vi "PicoScope4000aStartStreaming.vi"(0 "error in":errorcluster, 1 "handle in":i16, 4 "Enabled array":i16[](array[numeric]), 5 "Acquisition Settings":T1 {"Time Units" items=["Nanoseconds (ns)", "Microseconds (us)", "Milliseconds (ms)", "Seconds (s)"]; "Down-Sample Mode" items=["None", "Aggregate", "Decimate", "Average"]}) -> (6 "Channel A":i16[](array[numeric]), 7 "Channel E":i16[](array[numeric]), 8 "Channel B":i16[](array[numeric]), 9 "Channel F":i16[](array[numeric]), 10 "Channel C":i16[](array[numeric]), 11 "Channel G":i16[](array[numeric]), 12 "Channel D":i16[](array[numeric]), 13 "Channel H":i16[](array[numeric]), 14 "error out":errorcluster, 15 "handle out":i16, 18 "Sample Interval":u32)   [LabVIEW 2009]
doc: "This VI starts the oscilloscope streaming. It outputs arrays that will contain samples once PicoScope3000aGetStreamingValues.vi has returned."
uses:
  ps4000aWrap.dll
  PS4000a.dll
panel:
  out "Channel H Min":i16[](array[numeric])
  out "Channel G Min":i16[](array[numeric])
  out "Channel F Min":i16[](array[numeric])
  out "Channel E Min":i16[](array[numeric])
  out "Channel D Min":i16[](array[numeric])
  out "Channel C Min":i16[](array[numeric])
  out "Channel B Min":i16[](array[numeric])
  out "Channel A Min":i16[](array[numeric])
  # "Overview Buffer Size is the size of the temporary buffers used to\nstore data before returning it to the application."
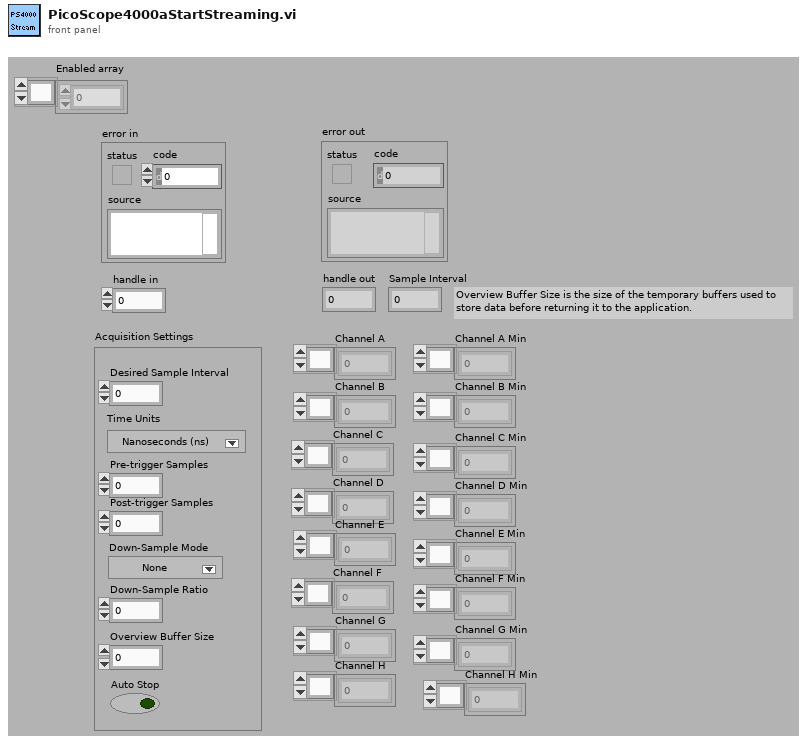
[diagram p1: front panel]
types:
  T1 = cluster{"Auto Stop":bool, "Desired Sample Interval":u32, "Pre-trigger Samples":u32, "Post-trigger Samples":u32, "Down-Sample Ratio":u32, "Down-Sample Mode":i32, "Overview Buffer Size":u32, "Time Units":u32}
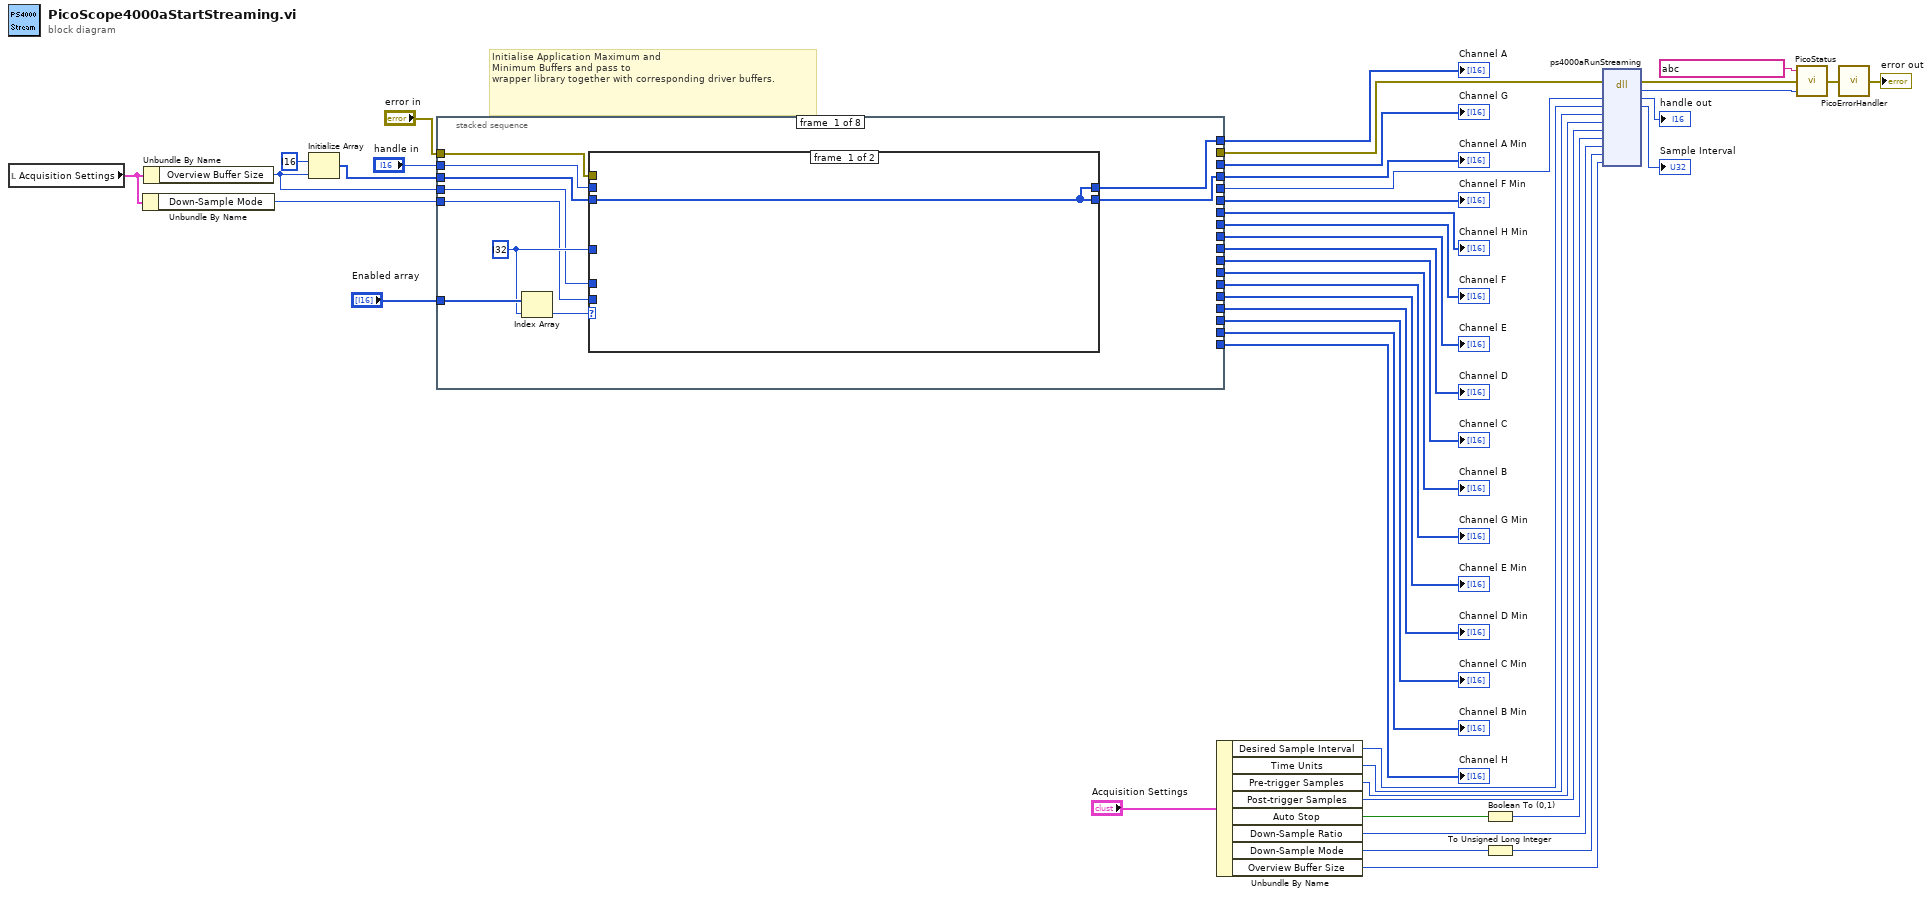
[diagram p0: block diagram]
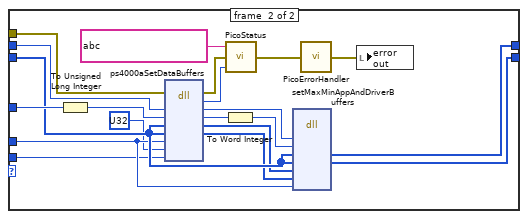
[diagram p2: hidden frame]
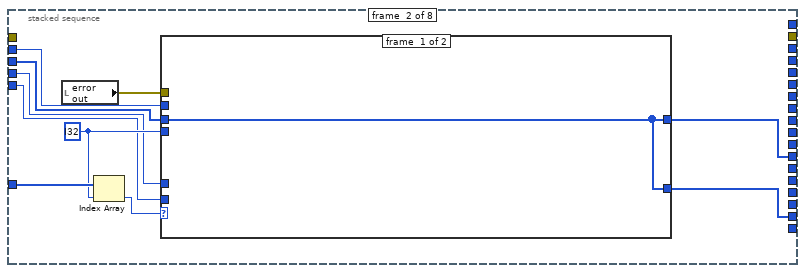
[diagram p3: hidden frame]
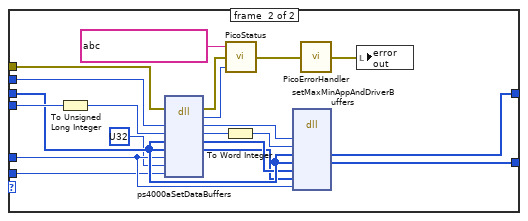
[diagram p4: hidden frame]
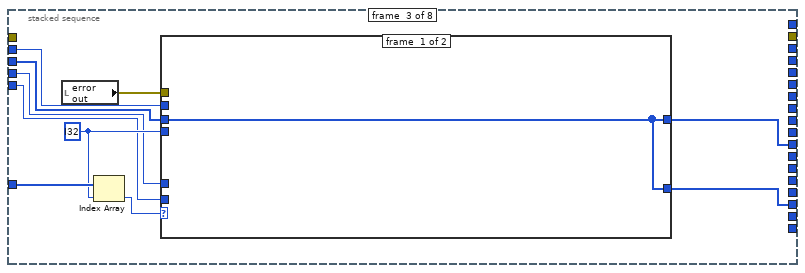
[diagram p5: hidden frame]
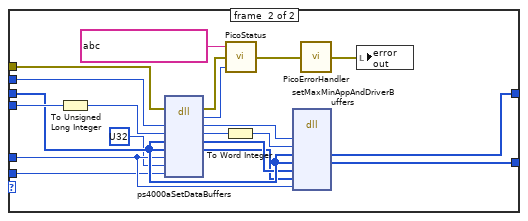
[diagram p6: hidden frame]
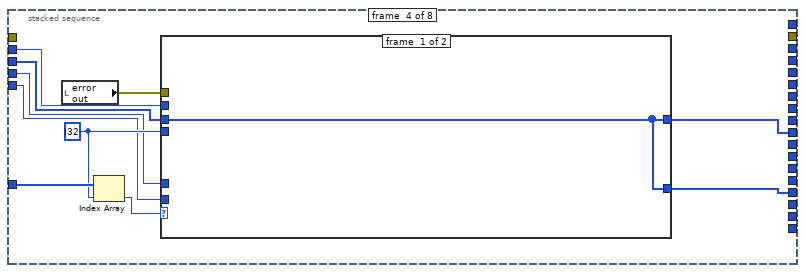
[diagram p7: hidden frame]
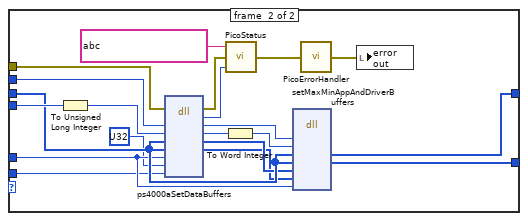
[diagram p8: hidden frame]
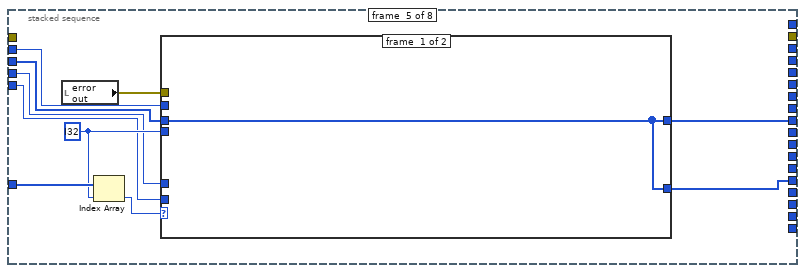
[diagram p9: hidden frame]
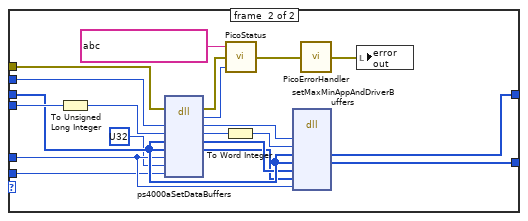
[diagram p10: hidden frame]
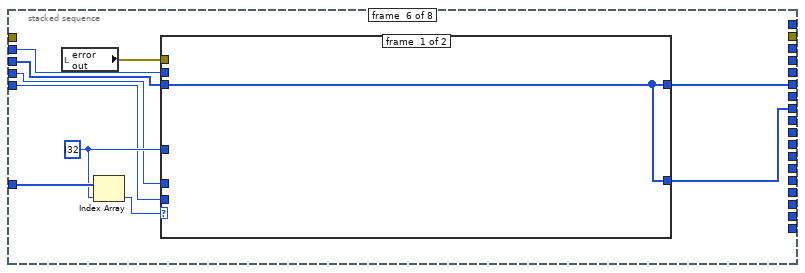
[diagram p11: hidden frame]
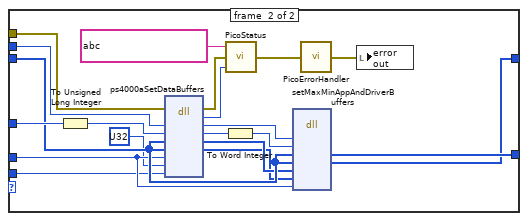
[diagram p12: hidden frame]
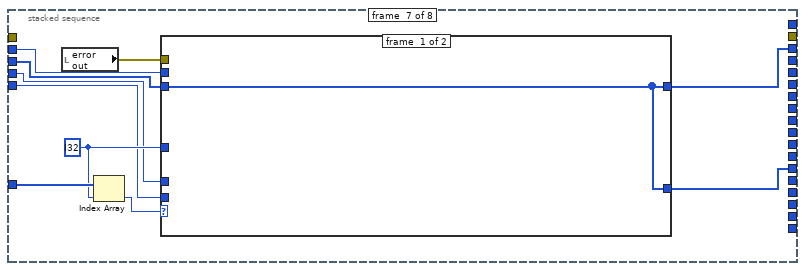
[diagram p13: hidden frame]
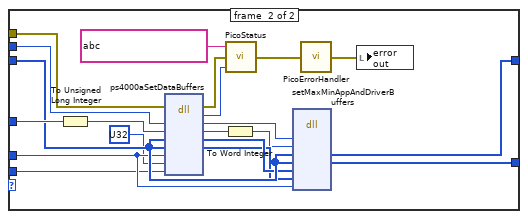
[diagram p14: hidden frame]
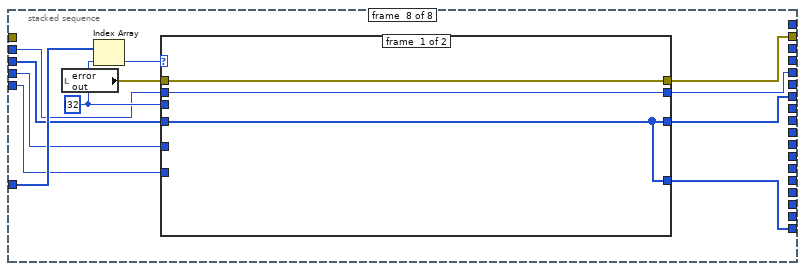
[diagram p15: hidden frame]
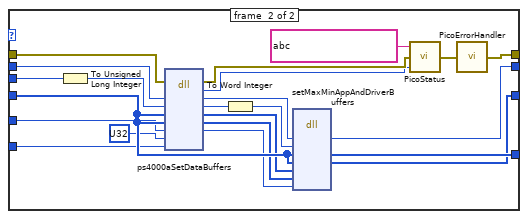
[diagram p16: hidden frame]
diagram:
  # "Initialise Application Maximum and\nMinimum Buffers and pass to \nwrapper library together with corresponding driver buffers."
  n1 = local read "Acquisition Settings"() -> (w31:T1)
  n2 = Unbundle By Name(w31) -> ("Down-Sample Mode"=w24:i32)
  n3 = Unbundle By Name(w31) -> ("Overview Buffer Size"=w22:u32)
  n4 = Initialize Array(i16 ? ("element"), w22) -> (w25:i16[])
  n5 = stacked-sequence {
    tunnel: "Enabled array" -> [w53 w84 w115 w146 w177 w208 w239 w272]
    tunnel: w25 -> [w51 w82 w113 w144 w175 w206 w237 w270]
    tunnel: "error in" -> [w50 _ _ _ _ _ _ _]
    tunnel: [w49 _ _ _ _ _ _ _] -> w16
    tunnel: [w48 _ _ _ _ _ _ _] -> w15
    tunnel: w22 -> [w47 w81 w112 w143 w174 w205 w236 w269]
    tunnel: w24 -> [w46 w80 w111 w142 w173 w204 w235 w268]
    tunnel: "handle in" -> [w45 w79 w110 w141 w172 w203 w234 w267]
    tunnel: [_ w78 _ _ _ _ _ _] -> w9
    tunnel: [_ w77 _ _ _ _ _ _] -> w14
    tunnel: [_ _ w108 _ _ _ _ _] -> w8
    tunnel: [_ _ w107 _ _ _ _ _] -> w13
    tunnel: [_ _ _ w139 _ _ _ _] -> w7
    tunnel: [_ _ _ w138 _ _ _ _] -> w11
    tunnel: [_ _ _ _ w170 _ _ _] -> w6
    tunnel: [_ _ _ _ w169 _ _ _] -> w12
    tunnel: [_ _ _ _ _ w201 _ _] -> w4
    tunnel: [_ _ _ _ _ w200 _ _] -> w5
    tunnel: [_ _ _ _ _ _ w232 _] -> w2
    tunnel: [_ _ _ _ _ _ w231 _] -> w3
    tunnel: [_ _ _ _ _ _ _ w265] -> w1
    tunnel: [_ _ _ _ _ _ _ w264] -> w10
    tunnel: [_ _ _ _ _ _ _ w263] -> w18
    tunnel: [_ _ _ _ _ _ _ w262] -> w17
    frame #0 {
      w52 = i32 ? ("index")
      n6 = Index Array(array=w53, index=w52) -> (element=w54:i16)
      n7 = case shown="1" w54 {
        tunnel: w52 -> [_ w75]
        tunnel: w51 -> [w55 w72]
        tunnel: w50 -> [_ w73]
        tunnel: [w55 w63] -> w49
        tunnel: [w55 w62] -> w48
        tunnel: w47 -> [_ w60]
        tunnel: w46 -> [_ w58]
        tunnel: w45 -> [_ w56]
        frame #0 {
        }
        frame #1 {
          n8 = To Unsigned Long Integer(number=w75) -> (unsigned 32bit integer=w74:u32)
          n9 = dll-call lib="PS4000a.dll" fn="ps4000aSetDataBuffers" ("ps3000.dll:_ps3000_open_unit@0")(error in=w73, "handle"=w56, "channel"=w74, "bufferMax"=w72, "bufferMin"=w72, "bufferLth"=w60, "segmentIndex"=u32 ?, "mode"=w58) -> (error out=w66:errorcluster, "PICO_STATUS"=w65:u32, "handle"=w69:i16, "channel"=w68:u32, "bufferMax"=w71:i16[], "bufferMin"=w70:i16[])  [unwired: 5 in, 1 out]
          n10 = To Word Integer(number=w68) -> (16bit integer=w67:i16)
          n11 = call "PicoStatus.vi"("PICO STATUS"=w65, "error in"=w66, "source"=string ?) -> ("error out"=w61:errorcluster)
          n12 = dll-call lib="ps4000aWrap.dll" fn="setMaxMinAppAndDriverBuffers" label="setMaxMinAppAndDriverBuffers\n(Channel A)"("handle"=w69, "channel"=w67, "appMaxBuffer"=w72, "appMinBuffer"=w72, "driverMaxBuffer"=w71, "driverMinBuffer"=w70, "bufferLength"=w60) -> ("appMaxBuffer"=w63:i16[], "appMinBuffer"=w62:i16[])  [unwired: 9 in, 2 out]
          n13 = call "PicoErrorHandler.vi"("error in"=w61) -> ("error out"=w57:errorcluster)
          n14 = local write "error out"(w57) -> ()
        }
      }
    }
    frame #1 {
      w83 = i32 ? ("index")
      n15 = local read "error out"() -> (w76:errorcluster)
      n16 = Index Array(array=w84, index=w83) -> (element=w85:i16)
      n17 = case shown="1" w85 {
        tunnel: w83 -> [_ w106]
        tunnel: w82 -> [w86 w103]
        tunnel: w76 -> [_ w104]
        tunnel: [w86 w94] -> w78
        tunnel: [w86 w93] -> w77
        tunnel: w81 -> [_ w91]
        tunnel: w80 -> [_ w89]
        tunnel: w79 -> [_ w87]
        frame #0 {
        }
        frame #1 {
          n18 = To Unsigned Long Integer(number=w106) -> (unsigned 32bit integer=w105:u32)
          n19 = dll-call lib="PS4000a.dll" fn="ps4000aSetDataBuffers" ("ps3000.dll:_ps3000_open_unit@0")(error in=w104, "handle"=w87, "channel"=w105, "bufferMax"=w103, "bufferMin"=w103, "bufferLth"=w91, "segmentIndex"=u32 ?, "mode"=w89) -> (error out=w97:errorcluster, "PICO_STATUS"=w96:u32, "handle"=w100:i16, "channel"=w99:u32, "bufferMax"=w102:i16[], "bufferMin"=w101:i16[])  [unwired: 5 in, 1 out]
          n20 = To Word Integer(number=w99) -> (16bit integer=w98:i16)
          n21 = call "PicoStatus.vi"("PICO STATUS"=w96, "error in"=w97, "source"=string ?) -> ("error out"=w92:errorcluster)
          n22 = dll-call lib="ps4000aWrap.dll" fn="setMaxMinAppAndDriverBuffers" label="setMaxMinAppAndDriverBuffers\n(Channel B)"("handle"=w100, "channel"=w98, "appMaxBuffer"=w103, "appMinBuffer"=w103, "driverMaxBuffer"=w102, "driverMinBuffer"=w101, "bufferLength"=w91) -> ("appMaxBuffer"=w94:i16[], "appMinBuffer"=w93:i16[])  [unwired: 9 in, 2 out]
          n23 = call "PicoErrorHandler.vi"("error in"=w92) -> ("error out"=w88:errorcluster)
          n24 = local write "error out"(w88) -> ()
        }
      }
    }
    frame #2 {
      w114 = i32 ? ("index")
      n25 = local read "error out"() -> (w109:errorcluster)
      n26 = Index Array(array=w115, index=w114) -> (element=w116:i16)
      n27 = case shown="1" w116 {
        tunnel: w114 -> [_ w137]
        tunnel: w113 -> [w117 w134]
        tunnel: w109 -> [_ w135]
        tunnel: [w117 w125] -> w108
        tunnel: [w117 w124] -> w107
        tunnel: w112 -> [_ w122]
        tunnel: w111 -> [_ w120]
        tunnel: w110 -> [_ w118]
        frame #0 {
        }
        frame #1 {
          n28 = To Unsigned Long Integer(number=w137) -> (unsigned 32bit integer=w136:u32)
          n29 = dll-call lib="PS4000a.dll" fn="ps4000aSetDataBuffers" ("ps3000.dll:_ps3000_open_unit@0")(error in=w135, "handle"=w118, "channel"=w136, "bufferMax"=w134, "bufferMin"=w134, "bufferLth"=w122, "segmentIndex"=u32 ?, "mode"=w120) -> (error out=w128:errorcluster, "PICO_STATUS"=w127:u32, "handle"=w131:i16, "channel"=w130:u32, "bufferMax"=w133:i16[], "bufferMin"=w132:i16[])  [unwired: 5 in, 1 out]
          n30 = To Word Integer(number=w130) -> (16bit integer=w129:i16)
          n31 = call "PicoStatus.vi"("PICO STATUS"=w127, "error in"=w128, "source"=string ?) -> ("error out"=w123:errorcluster)
          n32 = dll-call lib="ps4000aWrap.dll" fn="setMaxMinAppAndDriverBuffers" label="setMaxMinAppAndDriverBuffers\n(Channel C)"("handle"=w131, "channel"=w129, "appMaxBuffer"=w134, "appMinBuffer"=w134, "driverMaxBuffer"=w133, "driverMinBuffer"=w132, "bufferLength"=w122) -> ("appMaxBuffer"=w125:i16[], "appMinBuffer"=w124:i16[])  [unwired: 9 in, 2 out]
          n33 = call "PicoErrorHandler.vi"("error in"=w123) -> ("error out"=w119:errorcluster)
          n34 = local write "error out"(w119) -> ()
        }
      }
    }
    frame #3 {
      w145 = i32 ? ("index")
      n35 = local read "error out"() -> (w140:errorcluster)
      n36 = Index Array(array=w146, index=w145) -> (element=w147:i16)
      n37 = case shown="1" w147 {
        tunnel: w145 -> [_ w168]
        tunnel: w144 -> [w148 w165]
        tunnel: w140 -> [_ w166]
        tunnel: [w148 w156] -> w139
        tunnel: [w148 w155] -> w138
        tunnel: w143 -> [_ w153]
        tunnel: w142 -> [_ w151]
        tunnel: w141 -> [_ w149]
        frame #0 {
        }
        frame #1 {
          n38 = To Unsigned Long Integer(number=w168) -> (unsigned 32bit integer=w167:u32)
          n39 = dll-call lib="PS4000a.dll" fn="ps4000aSetDataBuffers" ("ps3000.dll:_ps3000_open_unit@0")(error in=w166, "handle"=w149, "channel"=w167, "bufferMax"=w165, "bufferMin"=w165, "bufferLth"=w153, "segmentIndex"=u32 ?, "mode"=w151) -> (error out=w159:errorcluster, "PICO_STATUS"=w158:u32, "handle"=w162:i16, "channel"=w161:u32, "bufferMax"=w164:i16[], "bufferMin"=w163:i16[])  [unwired: 5 in, 1 out]
          n40 = To Word Integer(number=w161) -> (16bit integer=w160:i16)
          n41 = call "PicoStatus.vi"("PICO STATUS"=w158, "error in"=w159, "source"=string ?) -> ("error out"=w154:errorcluster)
          n42 = dll-call lib="ps4000aWrap.dll" fn="setMaxMinAppAndDriverBuffers" label="setMaxMinAppAndDriverBuffers\n(Channel D)"("handle"=w162, "channel"=w160, "appMaxBuffer"=w165, "appMinBuffer"=w165, "driverMaxBuffer"=w164, "driverMinBuffer"=w163, "bufferLength"=w153) -> ("appMaxBuffer"=w156:i16[], "appMinBuffer"=w155:i16[])  [unwired: 9 in, 2 out]
          n43 = call "PicoErrorHandler.vi"("error in"=w154) -> ("error out"=w150:errorcluster)
          n44 = local write "error out"(w150) -> ()
        }
      }
    }
    frame #4 {
      w176 = i32 ? ("index")
      n45 = local read "error out"() -> (w171:errorcluster)
      n46 = Index Array(array=w177, index=w176) -> (element=w178:i16)
      n47 = case shown="1" w178 {
        tunnel: w176 -> [_ w199]
        tunnel: w175 -> [w179 w196]
        tunnel: w171 -> [_ w197]
        tunnel: [w179 w187] -> w170
        tunnel: [w179 w186] -> w169
        tunnel: w174 -> [_ w184]
        tunnel: w173 -> [_ w182]
        tunnel: w172 -> [_ w180]
        frame #0 {
        }
        frame #1 {
          n48 = To Unsigned Long Integer(number=w199) -> (unsigned 32bit integer=w198:u32)
          n49 = dll-call lib="PS4000a.dll" fn="ps4000aSetDataBuffers" ("ps3000.dll:_ps3000_open_unit@0")(error in=w197, "handle"=w180, "channel"=w198, "bufferMax"=w196, "bufferMin"=w196, "bufferLth"=w184, "segmentIndex"=u32 ?, "mode"=w182) -> (error out=w190:errorcluster, "PICO_STATUS"=w189:u32, "handle"=w193:i16, "channel"=w192:u32, "bufferMax"=w195:i16[], "bufferMin"=w194:i16[])  [unwired: 5 in, 1 out]
          n50 = To Word Integer(number=w192) -> (16bit integer=w191:i16)
          n51 = call "PicoStatus.vi"("PICO STATUS"=w189, "error in"=w190, "source"=string ?) -> ("error out"=w185:errorcluster)
          n52 = dll-call lib="ps4000aWrap.dll" fn="setMaxMinAppAndDriverBuffers" label="setMaxMinAppAndDriverBuffers\n(Channel E)"("handle"=w193, "channel"=w191, "appMaxBuffer"=w196, "appMinBuffer"=w196, "driverMaxBuffer"=w195, "driverMinBuffer"=w194, "bufferLength"=w184) -> ("appMaxBuffer"=w187:i16[], "appMinBuffer"=w186:i16[])  [unwired: 9 in, 2 out]
          n53 = call "PicoErrorHandler.vi"("error in"=w185) -> ("error out"=w181:errorcluster)
          n54 = local write "error out"(w181) -> ()
        }
      }
    }
    frame #5 {
      w207 = i32 ? ("index")
      n55 = local read "error out"() -> (w202:errorcluster)
      n56 = Index Array(array=w208, index=w207) -> (element=w209:i16)
      n57 = case shown="1" w209 {
        tunnel: w207 -> [_ w230]
        tunnel: w206 -> [w210 w227]
        tunnel: w202 -> [_ w228]
        tunnel: [w210 w218] -> w201
        tunnel: [w210 w217] -> w200
        tunnel: w205 -> [_ w215]
        tunnel: w204 -> [_ w213]
        tunnel: w203 -> [_ w211]
        frame #0 {
        }
        frame #1 {
          n58 = To Unsigned Long Integer(number=w230) -> (unsigned 32bit integer=w229:u32)
          n59 = dll-call lib="PS4000a.dll" fn="ps4000aSetDataBuffers" ("ps3000.dll:_ps3000_open_unit@0")(error in=w228, "handle"=w211, "channel"=w229, "bufferMax"=w227, "bufferMin"=w227, "bufferLth"=w215, "segmentIndex"=u32 ?, "mode"=w213) -> (error out=w221:errorcluster, "PICO_STATUS"=w220:u32, "handle"=w224:i16, "channel"=w223:u32, "bufferMax"=w226:i16[], "bufferMin"=w225:i16[])  [unwired: 5 in, 1 out]
          n60 = To Word Integer(number=w223) -> (16bit integer=w222:i16)
          n61 = call "PicoStatus.vi"("PICO STATUS"=w220, "error in"=w221, "source"=string ?) -> ("error out"=w216:errorcluster)
          n62 = dll-call lib="ps4000aWrap.dll" fn="setMaxMinAppAndDriverBuffers" label="setMaxMinAppAndDriverBuffers\n(Channel F)"("handle"=w224, "channel"=w222, "appMaxBuffer"=w227, "appMinBuffer"=w227, "driverMaxBuffer"=w226, "driverMinBuffer"=w225, "bufferLength"=w215) -> ("appMaxBuffer"=w218:i16[], "appMinBuffer"=w217:i16[])  [unwired: 9 in, 2 out]
          n63 = call "PicoErrorHandler.vi"("error in"=w216) -> ("error out"=w212:errorcluster)
          n64 = local write "error out"(w212) -> ()
        }
      }
    }
    frame #6 {
      w238 = i32 ? ("index")
      n65 = local read "error out"() -> (w233:errorcluster)
      n66 = Index Array(array=w239, index=w238) -> (element=w240:i16)
      n67 = case shown="1" w240 {
        tunnel: w238 -> [_ w261]
        tunnel: w237 -> [w241 w258]
        tunnel: w233 -> [_ w259]
        tunnel: [w241 w249] -> w232
        tunnel: [w241 w248] -> w231
        tunnel: w236 -> [_ w246]
        tunnel: w235 -> [_ w244]
        tunnel: w234 -> [_ w242]
        frame #0 {
        }
        frame #1 {
          n68 = To Unsigned Long Integer(number=w261) -> (unsigned 32bit integer=w260:u32)
          n69 = dll-call lib="PS4000a.dll" fn="ps4000aSetDataBuffers" ("ps3000.dll:_ps3000_open_unit@0")(error in=w259, "handle"=w242, "channel"=w260, "bufferMax"=w258, "bufferMin"=w258, "bufferLth"=w246, "segmentIndex"=u32 ?, "mode"=w244) -> (error out=w252:errorcluster, "PICO_STATUS"=w251:u32, "handle"=w255:i16, "channel"=w254:u32, "bufferMax"=w257:i16[], "bufferMin"=w256:i16[])  [unwired: 5 in, 1 out]
          n70 = To Word Integer(number=w254) -> (16bit integer=w253:i16)
          n71 = call "PicoStatus.vi"("PICO STATUS"=w251, "error in"=w252, "source"=string ?) -> ("error out"=w247:errorcluster)
          n72 = dll-call lib="ps4000aWrap.dll" fn="setMaxMinAppAndDriverBuffers" label="setMaxMinAppAndDriverBuffers\n(Channel G)"("handle"=w255, "channel"=w253, "appMaxBuffer"=w258, "appMinBuffer"=w258, "driverMaxBuffer"=w257, "driverMinBuffer"=w256, "bufferLength"=w246) -> ("appMaxBuffer"=w249:i16[], "appMinBuffer"=w248:i16[])  [unwired: 9 in, 2 out]
          n73 = call "PicoErrorHandler.vi"("error in"=w247) -> ("error out"=w243:errorcluster)
          n74 = local write "error out"(w243) -> ()
        }
      }
    }
    frame #7 {
      w271 = i32 ? ("index")
      n75 = local read "error out"() -> (w266:errorcluster)
      n76 = Index Array(array=w272, index=w271) -> (element=w273:i16)
      n77 = case shown="1" w273 {
        tunnel: w271 -> [_ w298]
        tunnel: w270 -> [w276 w295]
        tunnel: w266 -> [w275 w296]
        tunnel: [w276 w286] -> w265
        tunnel: [w276 w285] -> w264
        tunnel: w269 -> [_ w283]
        tunnel: w268 -> [_ w281]
        tunnel: w267 -> [w274 w280]
        tunnel: [w275 w279] -> w263
        tunnel: [w274 w278] -> w262
        frame #0 {
        }
        frame #1 {
          n78 = To Unsigned Long Integer(number=w298) -> (unsigned 32bit integer=w297:u32)
          n79 = dll-call lib="PS4000a.dll" fn="ps4000aSetDataBuffers" ("ps3000.dll:_ps3000_open_unit@0")(error in=w296, "handle"=w280, "channel"=w297, "bufferMax"=w295, "bufferMin"=w295, "bufferLth"=w283, "segmentIndex"=u32 ?, "mode"=w281) -> (error out=w289:errorcluster, "PICO_STATUS"=w288:u32, "handle"=w292:i16, "channel"=w291:u32, "bufferMax"=w294:i16[], "bufferMin"=w293:i16[], "bufferLth"=w277:i32)  [unwired: 4 in, 1 out]
          n80 = To Word Integer(number=w291) -> (16bit integer=w290:i16)
          n81 = dll-call lib="ps4000aWrap.dll" fn="setMaxMinAppAndDriverBuffers" label="setMaxMinAppAndDriverBuffers\n(Channel H)"("handle"=w292, "channel"=w290, "appMaxBuffer"=w295, "appMinBuffer"=w295, "driverMaxBuffer"=w294, "driverMinBuffer"=w293, "bufferLength"=w277) -> ("handle"=w278:i16, "appMaxBuffer"=w286:i16[], "appMinBuffer"=w285:i16[])  [unwired: 8 in, 2 out]
          n82 = call "PicoStatus.vi"("PICO STATUS"=w288, "error in"=w289, "source"=string ?) -> ("error out"=w284:errorcluster)
          n83 = call "PicoErrorHandler.vi"("error in"=w284) -> ("error out"=w279:errorcluster)
        }
      }
    }
  }
  "Channel A" <- w16
  "Channel A Min" <- w15
  "Channel B" <- w9
  "Channel B Min" <- w14
  "Channel C" <- w8
  "Channel C Min" <- w13
  "Channel D" <- w7
  "Channel D Min" <- w11
  "Channel E" <- w6
  "Channel E Min" <- w12
  "Channel F" <- w4
  "Channel F Min" <- w5
  "Channel G" <- w2
  "Channel G Min" <- w3
  "Channel H" <- w1
  "Channel H Min" <- w10
  n84 = Unbundle By Name("Acquisition Settings") -> ("Desired Sample Interval"=w38:u32, "Time Units"=w29:u32, "Pre-trigger Samples"=w37:u32, "Post-trigger Samples"=w36:u32, "Auto Stop"=w35:bool, "Down-Sample Ratio"=w33:u32, "Down-Sample Mode"=w32:i32, "Overview Buffer Size"=w30:u32)
  n85 = Boolean To (0,1)(Boolean=w35) -> (0, 1=w39:i16)
  n86 = To Unsigned Long Integer(number=w32) -> (unsigned 32bit integer=w28:u32)
  n87 = dll-call lib="ps4000A.dll" fn="ps4000aRunStreaming" ("ps5000a.dll:_ps3000_open_unit@0")(error in=w18, "handle"=w17, "sampleInterval"=w38, "sampleIntervalTimeUnits"=w29, "maxPreTriggerSamples"=w37, "maxPostTriggerSamples"=w36, "autoStop"=w39, "downSampleRatio"=w33, "downSampleRatioMode"=w28, "overviewBufferSize"=w30) -> (error out=w42:errorcluster, "PICO_STATUS"=w43:u32, "handle"=→"handle out":i16, "sampleInterval"=→"Sample Interval":u32)  [unwired: 9 in, 1 out]
  n88 = call "PicoStatus.vi"("PICO STATUS"=w43, "error in"=w42, "source"=string ?) -> ("error out"=w20:errorcluster)
  n89 = call "PicoErrorHandler.vi"("error in"=w20) -> ("error out"=→"error out":errorcluster)
